vi "red_tweezers_globals_INTERNAL.vi"() -> ()   [LabVIEW 2015]
doc: "This global contains settings used internally by Red Tweezers.\n\n\n(the line below ensures its settings are saved when necessary)"
uses:
  overlay_element.ctl
  <vilib>/Analysis/Matrix/Datatypes/RealMatrix.ctl
  <vilib>/Analysis/Matrix/NI_Matrix.lvlib
panel:
  in  "SLM 2D rotation and flipping":T1=[[1.0, 0.0, 0.0], [0.0, 1.0, 0.0], [0.0, 0.0, 1.0]]
  in  "SLM Transformation":T1=[[1.0, 0.0, 0.0], [0.0, 1.0, 0.0], [0.0, 0.0, 1.0]]
  in  "Zero Position On Camera/pixels":cluster{"X":dbl, "Y":dbl}={"X"=320.0, "Y"=240.0}
  in  "Display":T2(ring)=enum."Big Image"
  in  "Image Overlay (extras from control loop)":T3[](array[typedef]) {"Drawing Mode" items=["Frame", "Fill", "Highlight"]}
  in  "Camera Pixel Size/m":cluster{dbl, dbl}={1e-07, 1e-07}
  in  "Global ROI":i32[](array[numeric])=[0, 0, 640, 480]
  # "Warning: the controls in this global should be considered read-only.  They are set from the Settings VI (UDP Sender Generic), and it is that VI that's responsible for setting them up when settings are loaded from the XML file."
  # "This scales from pixels to metres- note that it should take account of magnification (e.g. a camera with 10um pixels, attached to a 100x microscope, has a pixel size of 100nm x 100nm)."
  # "This should be set to the position of the zero order spot (simplest way to set this is to create a trap at (0,0) and then adjust this to place the trap marker on top of the laser spot/a trapped object."
  # "The two transformation matrices here are applied to tweak \"real coordinates\" before they are used to generate spots on the SLM.  Typically, they flip rotate and (slightly) scale the spots.  These should ALWAYS be adjusted together.  The rotation and flipping one is the appropriate transform to apply to the NA coordinates (i.e. rotation in the XY plane and flipping of either X or Y)."
  # "The ROI sets the area of the camera that we use.  Normally this should be (0,0,width,height)\nwhere width and height are the vertical and horizontal resolution of your camera's sensor \n(in pixels)."
  # "This setting is in here for compatibility with the stereoscopic version of Red Tweezers.  It should be left set on \"mono image\"."
  # "This variable is used to add decorations to the image.  Points are given in the XY plane, but in REAL units.  This is set programatically, so you can safely ignore it here."
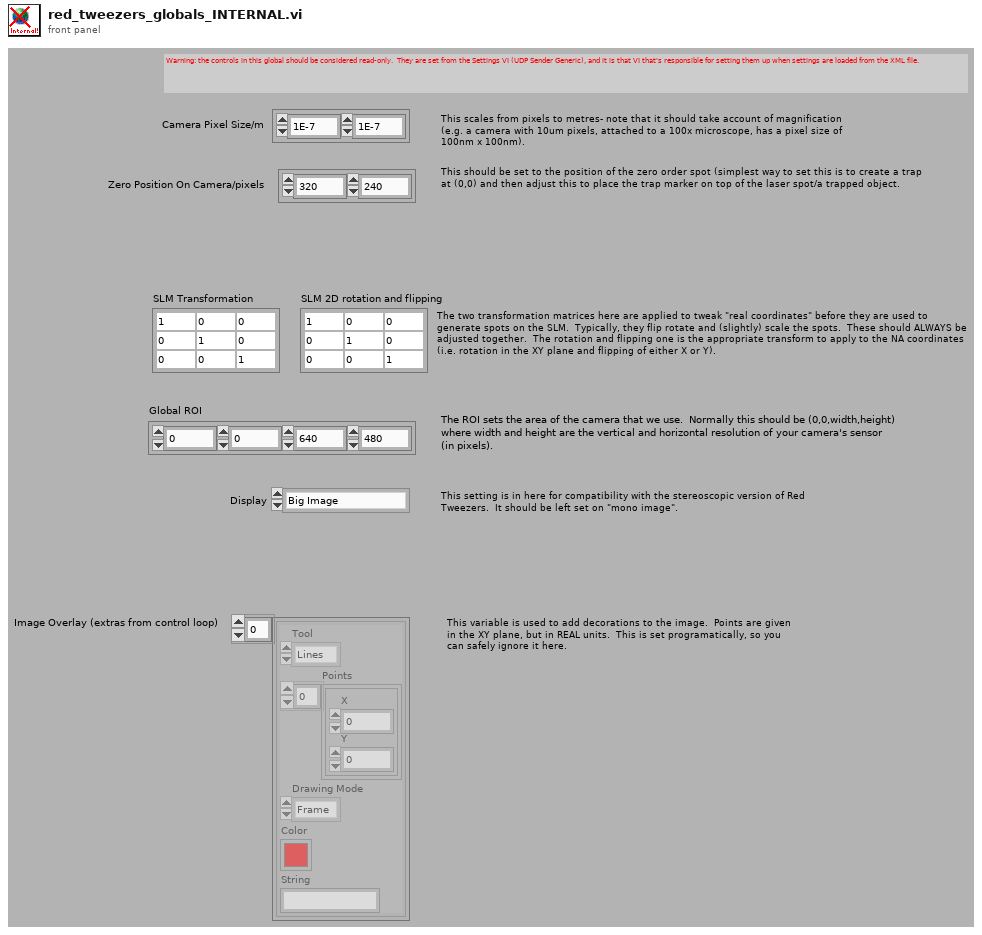
[diagram p1: front panel]
types:
  T1 = typedef "NI_Matrix.lvlib/RealMatrix.ctl" = dbl[][]
  T2 = enum16{"Left View", "Right View", "Big Image", "Anaglyph", "Side-By-Side", "None", "Mono Image"}
  T3 = typedef "overlay_element.ctl" = cluster{"Tool":enum16{"Lines", "Oval", "Rectangle", "Text"}, "Points":cluster{"X":dbl, "Y":dbl}[], "Drawing Mode":u32, "Color":u32, "String":string}
diagram:
